vi "Popup Message CORE.vi"(9 "Duration (s)":u32=6, 10 "Message Type":enum16{"INFO", "WARNING", "ERROR"}(ring), 11 "Message":string="Your Message Here.") -> ()   [LabVIEW 2011, in "COSYLib.lvlib"]
doc: "This VI provides a small popup notification window that fades in, displays a message, and fades out after a specified number of seconds."
uses:
  COSYLib.lvlib
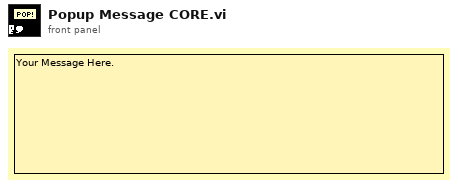
[diagram p1: front panel]
types:
  T1 = typedef "LVRectTypeDef.ctl" = cluster{"left":i16, "top":i16, "right":i16, "bottom":i16}
  T2 = typedef "eventvkey.ctl" = enum16{"ASCII", "Enter", "Return", "Shift", "Ctrl", "Alt", "Cmd", "Opt", "Caps", "NumLock", "Clear", "Break", "Up", "Down", "Left", "Right", "Insert", "Delete", "Home", "End", "PageUp", "PageDown", "Escape", "Help", "Pause", "ScrollLock", "F1", "F2", "F3", "F4", "F5", "F6", "F7", "F8", "F9", "F10", "F11", "F12", "F13", "F14", "F15", "F16", "F17", "F18", "F19", "F20", "F21", "F22", "F23", "F24", "Play", "VolumeUp", "VolumeDown", "Mute", "Two Byte Char"}
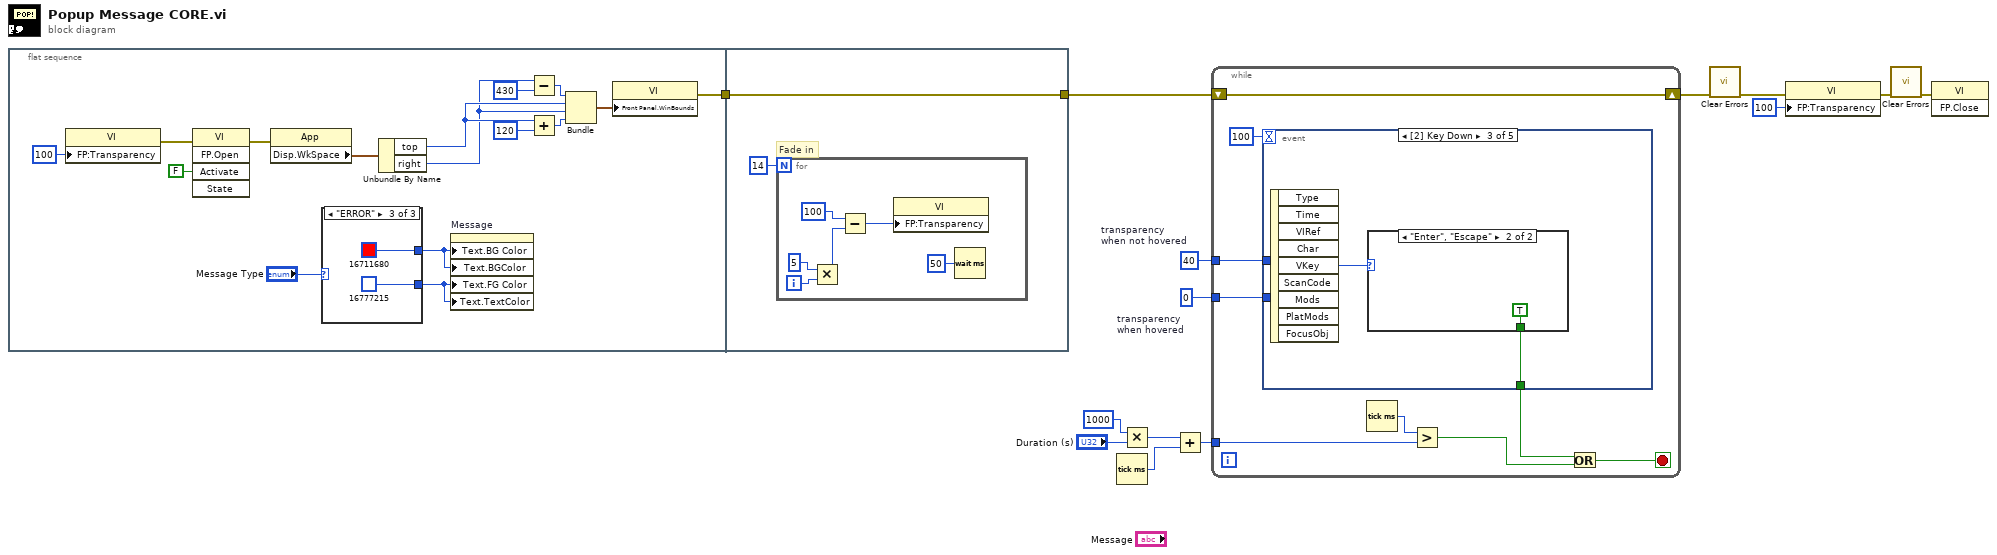
[diagram p0: block diagram]
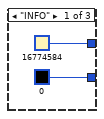
[diagram p2: hidden frame]
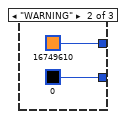
[diagram p3: hidden frame]
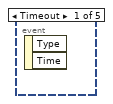
[diagram p4: hidden frame]
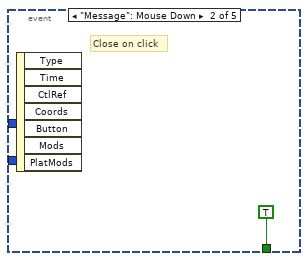
[diagram p5: hidden frame]
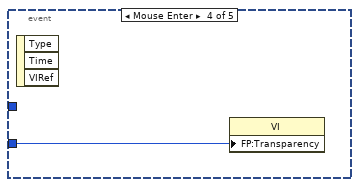
[diagram p7: hidden frame]
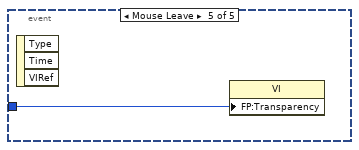
[diagram p8: hidden frame]
diagram:
  w6 = u8 0  # transparency when hovered
  w7 = u8 40  # transparency when not hovered
  n1 = flat-sequence {
    tunnel: [w22] -> w8
    tunnel: [w38] -> w11
    tunnel: w8 -> [w38]
    frame #0 {
      n2 = property class="VI"("FP:Transparency"=u8 100 ("Front Panel Window:Transparency")) -> (error out=w19:errorcluster)  [unwired: 2 in, 1 out]
      n3 = invoke class="VI" method="FP.Open"(error in=w19, "Activate"=FALSE ("Activate?")) -> (error out=w18:errorcluster)  [unwired: 3 in, 4 out]
      n4 = property class="App"(error in=w18) -> ("Disp.WkSpace"=w23:T1)  [unwired: 1 in, 2 out]
      n5 = case shown="\"ERROR\"" "Message Type" {
        tunnel: [u32 16774584 u32 16749610 u32 16711680] -> w16
        tunnel: [u32 0 u32 0 u32 16777215] -> w15
        frame "INFO" {
        }
        frame "WARNING" {
        }
        frame "ERROR" {
        }
      }
      n6 = Unbundle By Name(w23) -> ("top"=w29:i16, "right"=w26:i16)
      n7 = property on="Message" class="Str"("Text.BG Color"=w16, "Text.BGColor"=w16, "Text.FG Color"=w15, "Text.TextColor"=w15) -> ()  [unwired: 2 in, 2 out]
      n8 = Subtract(x=w26, y=i16 430) -> (x-y=w24:i16)
      n9 = Add(x=w29, y=i16 120) -> (x+y=w27:i16)
      n10 = Bundle(w24, "top"=w29, "right"=w26, w27) -> (w30:cluster{i16, "top":i16, "right":i16, i16})  [unwired: 1 in]
      n11 = property class="VI"("Front Panel.WinBounds"=w30) -> (error out=w22:errorcluster)  [unwired: 2 in, 1 out]
    }
    frame #1 {
      # "Fade in"
      n12 = for {
        N: 14 -> [_]
        i -> [w41]
        n13 = Multiply(x=5, y=w41) -> (x*y=w39:i32)
        n14 = Subtract(x=100, y=w39) -> (x-y=w43:i32)
        n15 = property class="VI"("FP:Transparency"=w43) -> ()  [unwired: 2 in, 2 out]
        n16 = Wait (ms)(milliseconds to wait=u32 50) -> ()  [unwired: 1 out]
      }
    }
  }
  n17 = Tick Count (ms)() -> (millisecond timer value=w13:u32)
  n18 = Multiply(x=u32 1000 ("y"), y="Duration (s)") -> (x*y=w10:u32)
  n19 = Add(x=w10, y=w13) -> (x+y=w12:u32)
  n20 = while {
    tunnel: w12 -> [w51]
    shift-right: [w47] -> w5
    shift-left: w11 -> [w47]
    tunnel: w7 -> [w46]
    tunnel: w6 -> [w45]
    stop <- w49 stop-if-true
    n21 = event shown="[2] Key Down" {
      selector: _ -> [_ _ _ _ _]
      dyn-events: _ -> [_ _ _ _ _]
      timeout: 100 -> [_ _ _ _ _]
      tunnel: [_ TRUE w55 _ _] -> w53
      tunnel: w46 -> [_ _ _ _ w59]
      tunnel: w45 -> [_ _ _ w58 _]
      event Timeout {
        n22 = event-data() -> ()  [unwired: 1 in, 2 out]
      }
      event "Message": Mouse Down {
        # "Close on click"
        n23 = event-data() -> ()  [unwired: 1 in, 7 out]
      }
      event Key Down {
        n24 = event-data() -> ("VKey"=w56:T2)  [unwired: 1 in, 8 out]
        n25 = case shown="\"Enter\", \"Escape\"" w56 {
          tunnel: [_ TRUE] -> w55
          frame Default {
          }
          frame "Enter", "Escape" {
          }
        }
      }
      event Mouse Enter {
        n26 = event-data() -> ()  [unwired: 1 in, 3 out]
        n27 = property class="VI"("FP:Transparency"=w58) -> ()  [unwired: 2 in, 2 out]
      }
      event Mouse Leave {
        n28 = event-data() -> ()  [unwired: 1 in, 3 out]
        n29 = property class="VI"("FP:Transparency"=w59) -> ()  [unwired: 2 in, 2 out]
      }
    }
    n30 = Tick Count (ms)() -> (millisecond timer value=w52:u32)
    n31 = Greater?(x=w52, y=w51) -> (0:w50:bool)
    n32 = Or(x=w53, y=w50) -> (x .or. y?=w49:bool)
  }
  n33 = call <vilib>:"Clear Errors.vi"("error in (no error)"=w5) -> ("error out"=w4:errorcluster)  [unwired: 6 in]
  n34 = property class="VI"(error in=w4, "FP:Transparency"=u8 100 ("Front Panel Window:Transparency")) -> (error out=w3:errorcluster)  [unwired: 1 in, 1 out]
  n35 = call <vilib>:"Clear Errors.vi"("error in (no error)"=w3) -> ("error out"=w1:errorcluster)  [unwired: 6 in]
  n36 = invoke class="VI" method="FP.Close"(error in=w1) -> ()  [unwired: 2 in, 3 out]
